vi "Available AI.vi"(8 "error in (no error)":errorcluster, 11 "DeviceComms in":refnum<class "DeviceComms.lvclass">) -> (0 "error out":errorcluster, 2 "Available AI":T1[](array[typedef]), 3 "DeviceComms out":refnum<class "DeviceComms.lvclass">)   [LabVIEW 2024, in "CTI.lvlib" / "DeviceComms.lvclass"]
uses:
  DeviceComms.lvclass
  Available AI.ctl
  ADC Number.ctl
  GPIO Number.ctl
  CTI.lvlib
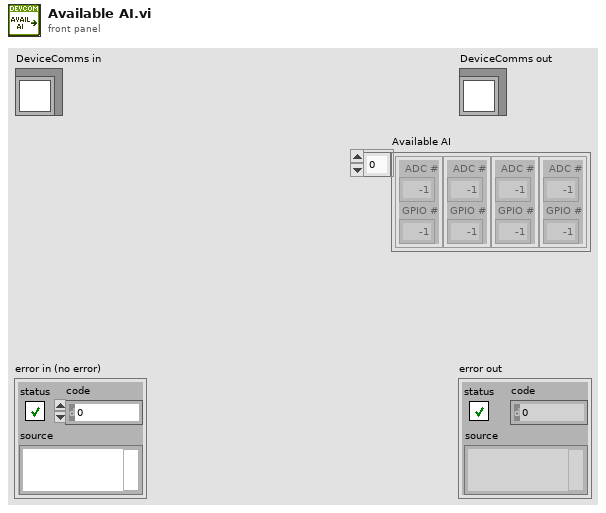
[diagram p1: front panel]
types:
  T1 = typedef "CTI.lvlib/Available AI.ctl" = cluster{"ADC #":T2, "GPIO #":T3}
  T2 = typedef "CTI.lvlib/ADC Number.ctl" = i8
  T3 = typedef "CTI.lvlib/GPIO Number.ctl" = i8
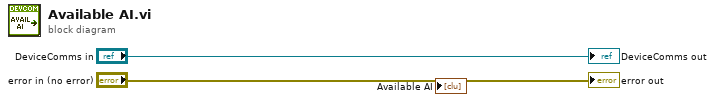
[diagram p0: block diagram]
diagram:
  "error out" <- "error in (no error)"
  "DeviceComms out" <- "DeviceComms in"
